vi "MultiAxisControl.vi"() -> ()   [LabVIEW 2018, in "Aerotech.lvlib"]
uses:
  Aerotech.lvlib
  Parameters/GetAxisParameterDouble.vi
  Motion/AbortSingle.vi
  Parameters/GetAxisParameterString.vi
  Motion/MoveIncSingle.vi
  Motion/FreerunSingle.vi
  Motion/FaultAckSingle.vi
  Motion/HomeSingle.vi
  Motion/DisableSingle.vi
  Motion/EnableSingle.vi
  Utility/AxisControl.ctl
panel:
  in  "Disconnect?":bool
  in  "Show First":i32=2 caption="Axes" min=0 max=32
  out "Status":string
  in  "StopProgram":bool caption="Stop"
  out "do stop":bool
  in  "stop":bool
  out "Error":string
  in  "Init":bool=TRUE
  in  "Abort Motion":bool
  in  "Reset Controller":bool
  in  "In Task:":i32(ring)=1 items=["TLibrary", "T01", "T02", "T03", "T04", "T05", "T06", "T07", "T08", "T09", "T10", "T11", "T12", "T13", "T14", "T15", "T16", "T17", "T18", "T19", "T20", "T21", "T22", "T23", "T24", "T25", "T26", "T27", "T28", "T29", "T30", "T31"]
  in  "ExecuteProgram":bool caption="Execute"
  in  "Program:":path
  in  "Axes":T1[](array[typedef])
  in  "Status":string
  in  "Execute":bool
  in  "Command:":string
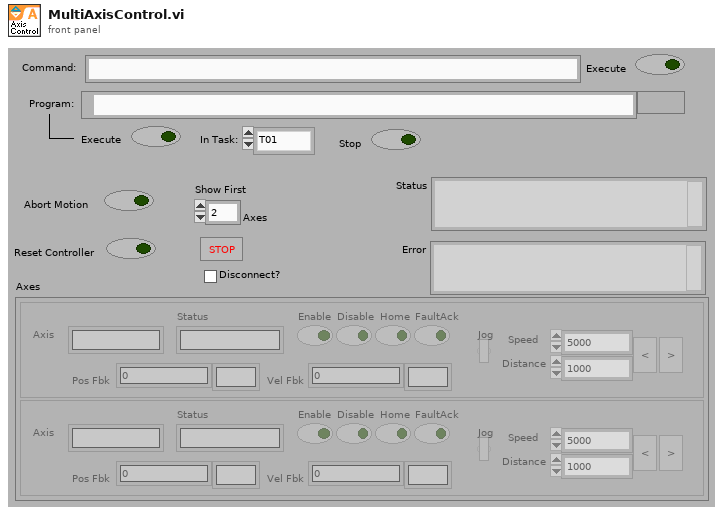
[diagram p1: front panel]
types:
  T1 = typedef "Aerotech.lvlib/AxisControl.ctl" = cluster{"Axis":string, "Enable":bool, "Disable":bool, "Home":bool, "FaultAck":bool, "Jog":bool, "Speed":dbl, "Distance":dbl, "Jog Left":bool, "Jog Right":bool, "Status":string, "Pos Fbk":dbl, "Vel Fbk":dbl, "Pos Units":string, "Vel Units":string}
  T2 = cluster{"new reference":refnum<k24>, "Event Callback":refnum<k27>, "ControllerDiagPacket":refnum<user-event>, "Event Registration Refnum":refnum<event-registration>}
  T3 = enum32{"invalid app kind", "Development System", "Run Time System", "Student Edition", "Embedded LabVIEW", "Evaluation", "Custom"}
  T4 = cluster{"Axis":string, "Enable":bool, "Disable":bool, "Home":bool, "FaultAck":bool, "Jog":bool, "Speed":dbl, "Distance":dbl, "Jog Left":bool, "Jog Right":bool, "Status":string, "Pos Fbk":dbl, "Vel Fbk":dbl, "Pos Units":string, "Vel Units":string}
  T5 = typedef "AxisDiagPacket.ctl" = cluster{"Axis Name":string, "Analog Input 0":dbl, "Analog Input 1":dbl, "Axis Fault (num)":i32, "Axis Fault (str)":string, "Axis Fault (bits)":cluster{"AmplifierFault":bool, "AmplifierTemperatureFault":bool, "CcwEndOfTravelLimitFault":bool, "CcwSoftwareLimitFault":bool, "CommunicationLostFault":bool, "CwEndOfTravelLimitFault":bool, "CwSoftwareLimitFault":bool, "EmergencyStopFault":bool, "EncoderFault":bool, "ExternalFault":bool, "FeedbackScalingFault":bool, "GantryMisalignFault ":bool, "HallSensorFault":bool, "InPositionTimeoutFault":bool, "MarkerSearchFault":bool, "MaxVelocityCommandFault":bool, "MissedInterruptFault":bool, "MotorTemperatureFault":bool, "None":bool, "OverCurrentFault":bool, "PositionErrorFault":bool, "PositionFeedbackFault":bool, "PowerSupplyFault":bool, "ProbeInputFault":bool, "SafeZoneFault":bool, "VelocityErrorFault":bool, "VelocityFeedbackFault":bool, "VoltageClampFault":bool, "InternalFault":bool}, "Axis Status (num)":i32, "Axis Status (str)":string, "Axis Status (bits)":cluster{"BacklashActive":bool, "CalibrationEnabled1D":bool, "CalibrationEnabled2D":bool, "CommandValid":bool, "DriveAbortPending":bool, "DrivePending":bool, "Enabling":bool, "GainMappingEnabled":bool, "GantryAligned":bool, "GantryRealigning":bool, "Homed":bool, "Homing":bool, "IFOVEnabled":bool, "JogGenerating":bool, "Jogging":bool, "JoystickControl":bool, "MasterSlaveControl":bool, "MotionBlocked":bool, "MotionClamped":bool, "MoveDone":bool, "None":bool, "NotVirtual":bool, "Profiling":bool, "Stability0":bool, "Stability1":bool, "TrajectoryFiltering":bool, "WaitDone":bool}, "Current Command":sgl, "Current Error":sgl, "Current Feedback":sgl, "Digital Inputs":i32, "Digital Outputs":i32, "Drive Status":i32, "Drive Status (str)":string, "Drive Status (bits)":cluster{"AccelerationPhase":bool, "AutofocusActive":bool, "BrakeOutput":bool, "CcwEndOfTravelLimitInput":bool, "CosineEncoderError":bool, "CurrentClamp":bool, "CwEndOfTravelLimitInput":bool, "DecelerationPhase":bool, "DualLoopActive":bool, "EmergencyStopInput":bool, "Enabled":bool, "EncoderClipping":bool, "GalvoCalibrationEnabled":bool, "GalvoPowerCorrection":bool, "HallAInput":bool, "HallBInput":bool, "HallCInput":bool, "HighResolutionMode":bool, "HomeLimitInput":bool, "InPosition":bool, "InPosition2":bool, "MarkerInput":bool, "MarkerLatch":bool, "MoveActive":bool, "NoMotorSupply":bool, "None":bool, "PowerLimiting":bool, "ProgrammingFlash":bool, "ProgrammingMXH":bool, "PSOHaltLatch":bool, "ServoControl":bool, "SineEncoderError":bool}, "Position Feedback Auxiliary":dbl, "Position Command":dbl, "Position Error":dbl, "Position Feedback":dbl, "Program Position Command":dbl, "Program Position Error":dbl, "Program Position Feedback":dbl, "Velocity Command":dbl, "Velocity Error":dbl, "Velocity Feedback":dbl}
  T6 = cluster{"Axis":string, "Enable":bool, "Disable":bool, "Home":bool, "FaultAck":bool, "Jog":bool, "Speed":dbl, "Distance":dbl, "Jog Left":bool, "Jog Right":bool, "Status":string, "Pos Fbk":dbl, "Vel Fbk":dbl, "Pos Units":string, "Vel Units":string}[]
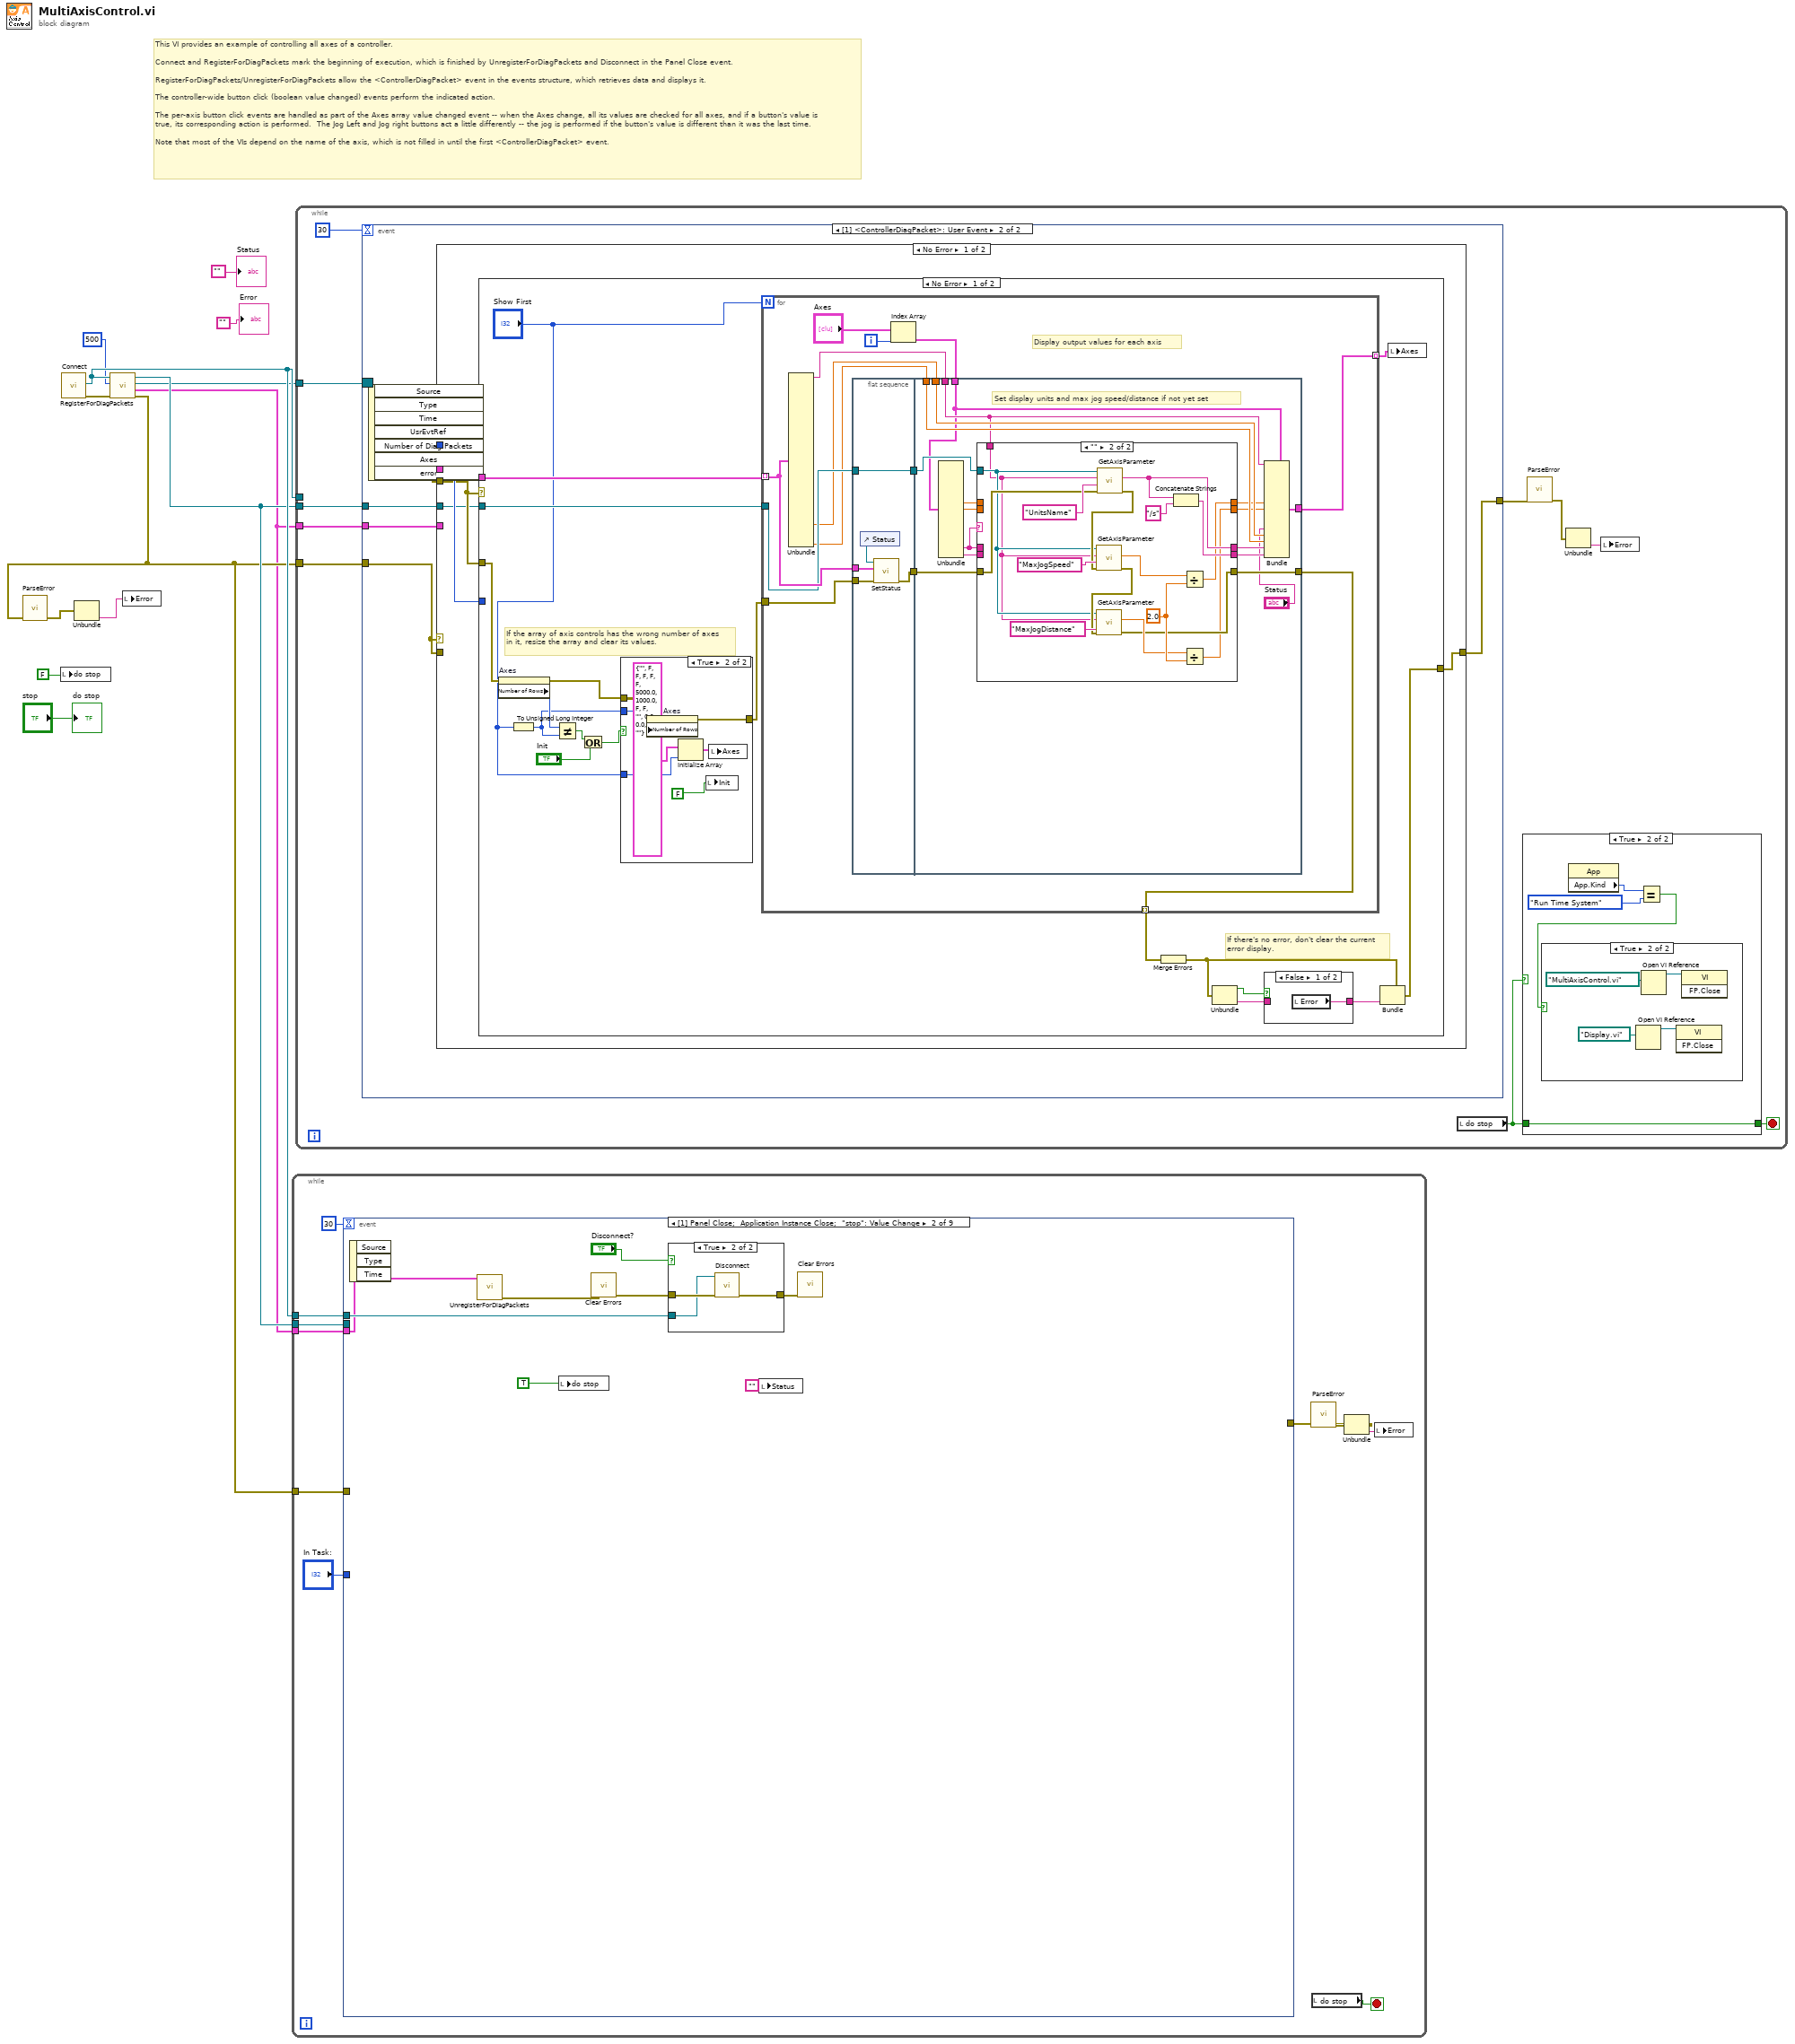
[diagram p0: block diagram]
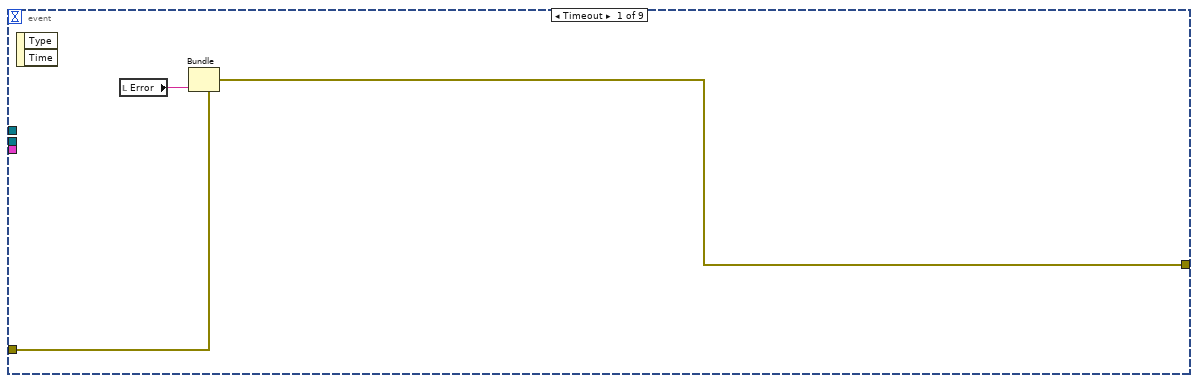
[diagram p2: hidden frame]
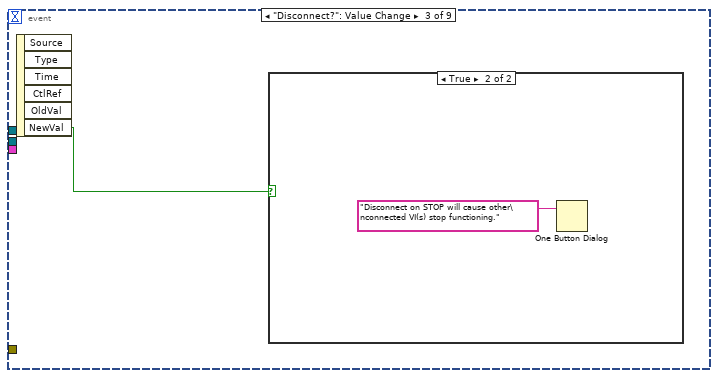
[diagram p4: hidden frame]
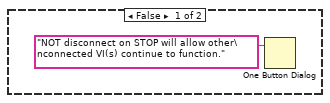
[diagram p5: hidden frame]
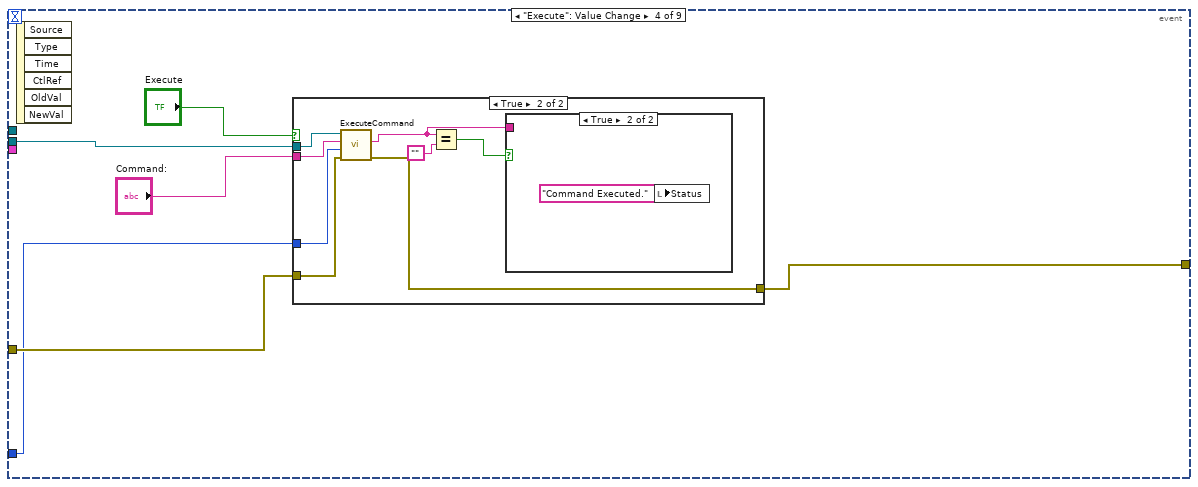
[diagram p6: hidden frame]
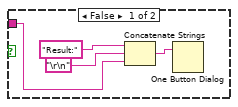
[diagram p8: hidden frame]
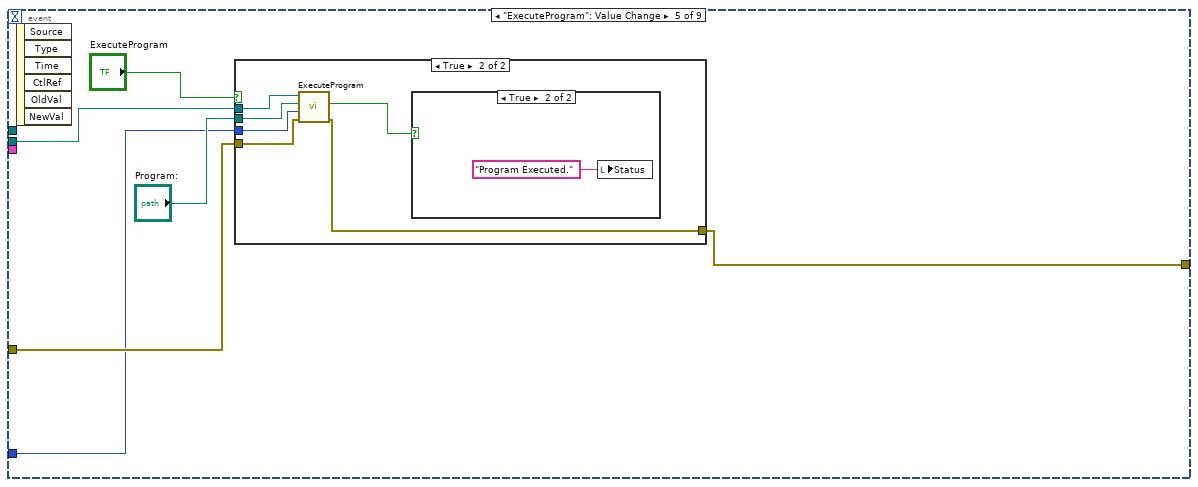
[diagram p9: hidden frame]
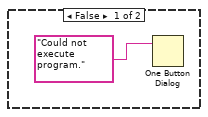
[diagram p11: hidden frame]
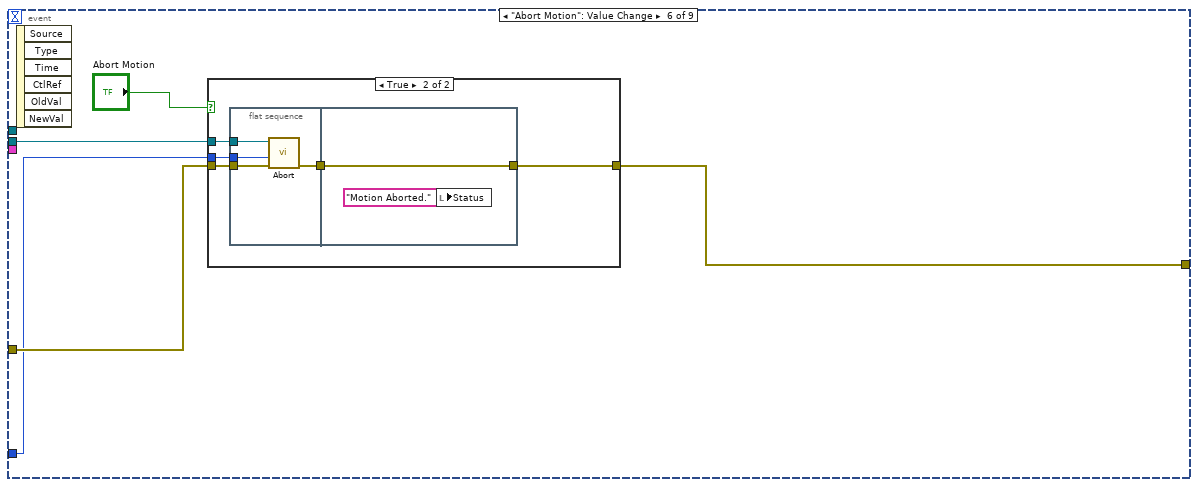
[diagram p12: hidden frame]
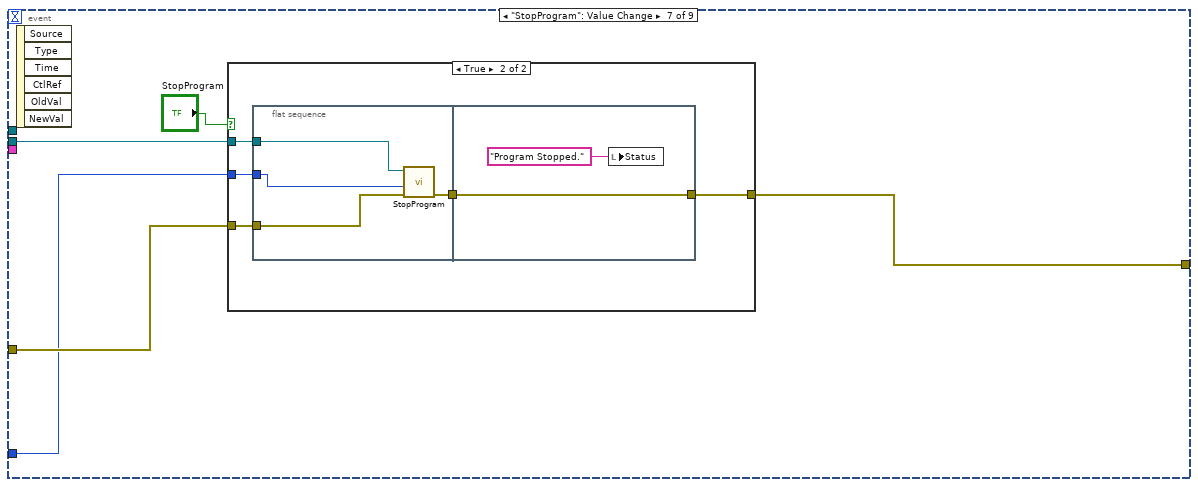
[diagram p14: hidden frame]
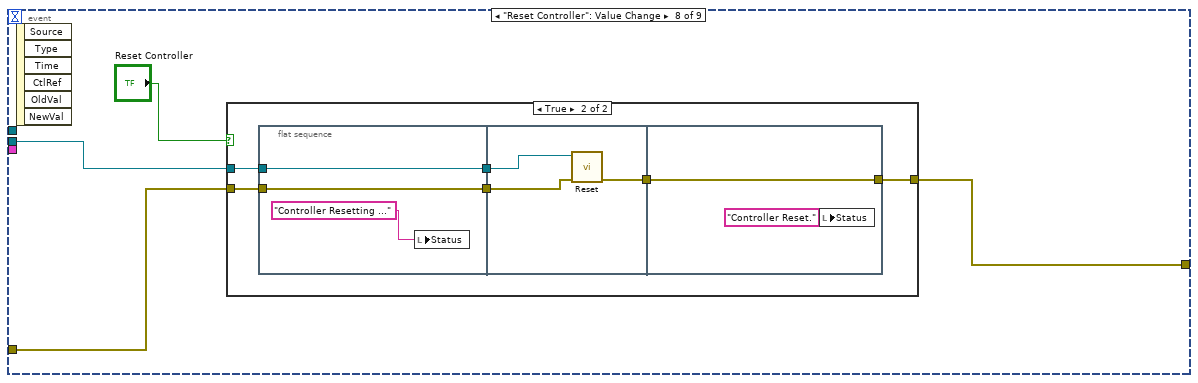
[diagram p16: hidden frame]
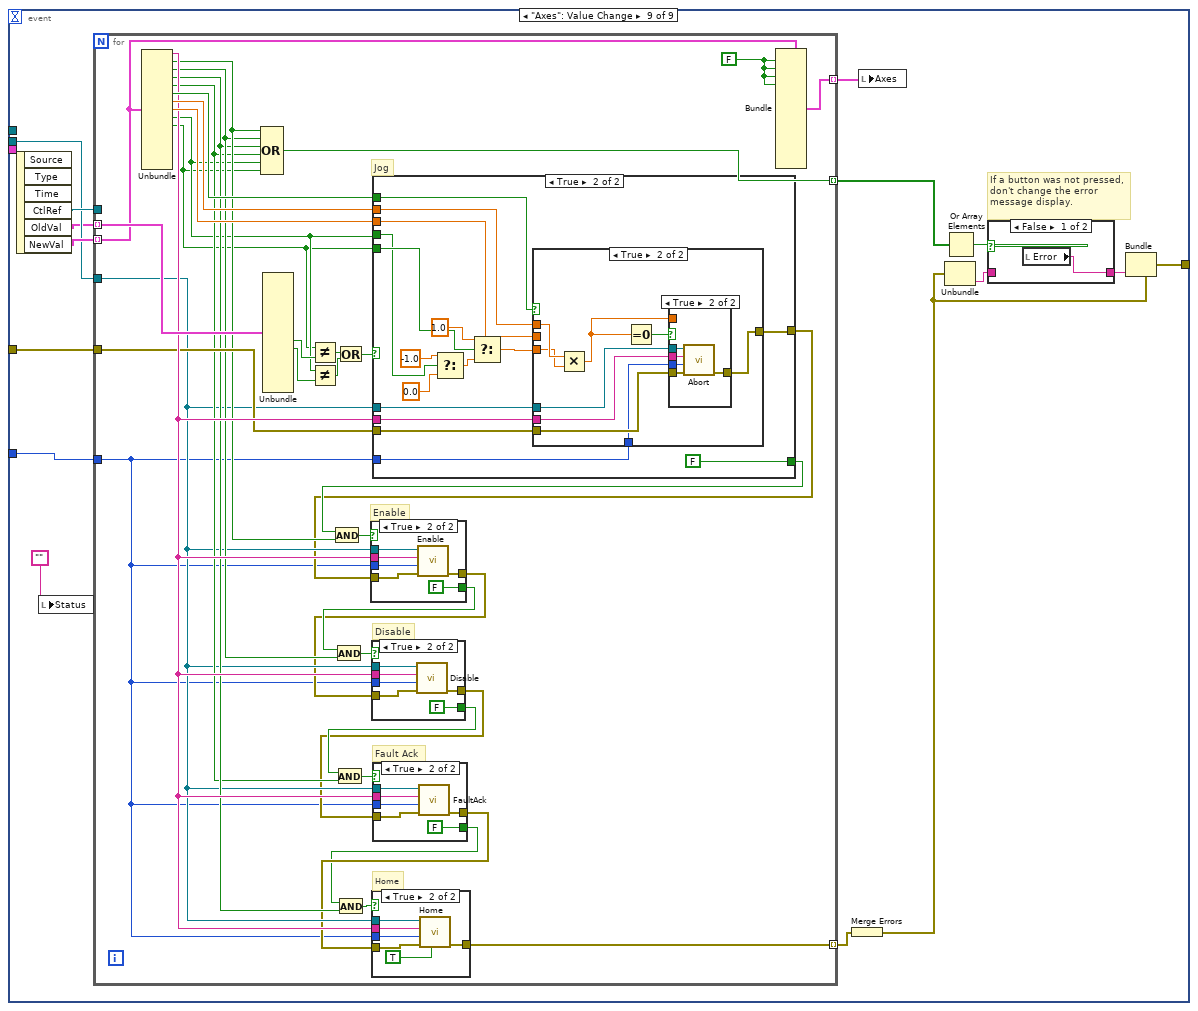
[diagram p18: hidden frame]
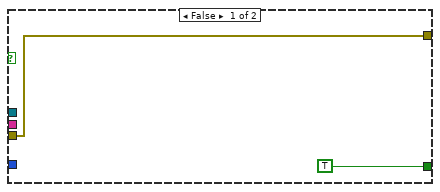
[diagram p20: hidden frame]
diagram:
  # "This VI provides an example of controlling all axes of a controller. \n\nConnect and RegisterForDiagPackets mark the beginning of execution, which is finished by UnregisterForDiagPackets and Disconnect in the Panel Close event.\n\nRegisterForDiagPackets/UnregisterForDiagPackets allow the <ControllerDiagPacket> event in the events structure, which retrieves data and displays it.\n\nThe controller-wide button click (boolean value changed) events perform the indicated action.\n\nThe per-axis button click events are handled as part of the Axes array value changed event -- when the Axes change, all its values are checked for all axes, and if a button's value is true, its corresponding action is performed.  The Jog Left and Jog right buttons act a little differently -- the jog is performed if the button's value is different than it was the last time.\n\nNote that most of the VIs depend on the name of the axis, which is not filled in until the first <ControllerDiagPacket> event."
  n1 = local write "do stop"(FALSE ("do stop")) -> ()
  n2 = call "Connect.vi"() -> ("error out"=w7:errorcluster, "controller"=w6:refnum<k24>)  [unwired: 10 in]
  n3 = call "RegisterForDiagPackets.vi"("error in (no error)"=w7, "refresh interval (default)"=500, "Controller in"=w6) -> ("error out"=w3:errorcluster, "Event Metadata"=w2:T2, "Event Registration Refnum"=w4:refnum<event-registration>, "Controller out"=w5:refnum<k24>)  [unwired: 4 in]
  n4 = call "ParseError.vi"("error in (no error)"=w3) -> ("error out"=w11:errorcluster)  [unwired: 10 in]
  n5 = Unbundle(w11) -> ("source"=w12:string)  [unwired: 2 out]
  n6 = local write "Error"(w12) -> ()
  n7 = while {
    tunnel: w6 -> [w19]
    tunnel: w5 -> [w18]
    tunnel: w3 -> [w17]
    tunnel: w2 -> [w14]
    stop <- w16 stop-if-true
    n8 = event shown="[1] Panel Close;  Application Instance Close;  \"stop\": Value Change" {
      selector: _ -> [_ _ _ _ _ _ _ _ _]
      dyn-events: _ -> [_ _ _ _ _ _ _ _ _]
      timeout: 30 -> [_ _ _ _ _ _ _ _ _]
      tunnel: w18 -> [_ _ _ w46 w66 w80 w95 w113 w142]
      tunnel: w17 -> [w26 _ _ w45 w64 w81 w97 w112 w141]
      tunnel: [w25 _ _ w43 w63 w78 w96 w111 w136] -> w21
      tunnel: w19 -> [_ w33 _ _ _ _ _ _ _]
      tunnel: "In Task:" -> [_ _ _ w42 w62 w77 w94 _ w130]
      tunnel: w14 -> [_ w27 _ _ _ _ _ _ _]
      event Timeout {
        n9 = event-data() -> ()  [unwired: 1 in, 2 out]
        n10 = local read "Error"() -> (w24:string)
        n11 = Bundle(cluster=w26, "source"=w24) -> (w25:errorcluster)  [unwired: 2 in]
      }
      event Panel Close; Application Instance Close; "stop": Value Change {
        n12 = event-data() -> ()  [unwired: 1 in, 3 out]
        n13 = call "UnregisterForDiagPackets.vi"("Event Metadata"=w27) -> ("error out"=w28:errorcluster)  [unwired: 9 in]
        n14 = local write "do stop"(TRUE) -> ()
        n15 = call <vilib>:"Clear Errors.vi"("error in (no error)"=w28) -> ("error out"=w34:errorcluster)  [unwired: 5 in, 1 out]
        n16 = case shown="True" "Disconnect?" {
          tunnel: w34 -> [w35 w38]
          tunnel: w33 -> [_ w37]
          tunnel: [w35 w36] -> w32
          frame False {
          }
          frame True {
            n17 = call "Disconnect.vi"("error in (no error)"=w38, "controller"=w37) -> ("error out"=w36:errorcluster)  [unwired: 9 in]
          }
        }
        n18 = local write "Status"("") -> ()
        n19 = call <vilib>:"Clear Errors.vi"("error in (no error)"=w32) -> ()  [unwired: 5 in, 2 out]
      }
      event "Disconnect?": Value Change {
        n20 = event-data() -> ("NewVal"=w39:bool)  [unwired: 1 in, 5 out]
        n21 = case shown="True" w39 {
          frame False {
            n22 = One Button Dialog(message="NOT disconnect on STOP will allow other\nconnected VI(s) continue to function.") -> ()  [unwired: 1 in, 1 out]
          }
          frame True {
            n23 = One Button Dialog(message="Disconnect on STOP will cause other\nconnected VI(s) stop functioning.") -> ()  [unwired: 1 in, 1 out]
          }
        }
      }
      event "Execute": Value Change {
        n24 = event-data() -> ()  [unwired: 1 in, 6 out]
        n25 = case shown="True" "Execute" {
          tunnel: w46 -> [_ w56]
          tunnel: w45 -> [w48 w54]
          tunnel: "Command:" -> [_ w55]
          tunnel: [w48 w50] -> w43
          tunnel: w42 -> [_ w49]
          frame False {
          }
          frame True {
            n26 = call "ExecuteCommand.vi"("error in (no error)"=w54, "taskId"=w49, "Command Code"=w55, "controller in"=w56) -> ("error out"=w50:errorcluster, "return value"=w51:string)  [unwired: 5 in, 1 out]
            n27 = Equal?(x=w51, y="") -> (x = y?=w52:bool)
            n28 = case shown="True" w52 {
              tunnel: w51 -> [w57 _]
              frame False {
                n29 = Concatenate Strings("Result:", "\r\n", w57) -> (w60:string)
                n30 = One Button Dialog(message=w60) -> ()  [unwired: 1 in, 1 out]
              }
              frame True {
                n31 = local write "Status"("Command Executed." ("Status")) -> ()
              }
            }
          }
        }
      }
      event "ExecuteProgram": Value Change {
        n32 = event-data() -> ()  [unwired: 1 in, 6 out]
        n33 = case shown="True" "ExecuteProgram" {
          tunnel: w66 -> [_ w74]
          tunnel: w64 -> [w68 w72]
          tunnel: "Program:" -> [_ w73]
          tunnel: w62 -> [_ w70]
          tunnel: [w68 w69] -> w63
          frame False {
          }
          frame True {
            n34 = call "ExecuteProgram.vi"("error in (no error)"=w72, "taskId"=w70, "program name and path"=w73, "controller in"=w74) -> ("error out"=w69:errorcluster, "success"=w71:bool)  [unwired: 5 in, 1 out]
            n35 = case shown="True" w71 {
              frame False {
                n36 = One Button Dialog(message="Could not execute program.") -> ()  [unwired: 1 in, 1 out]
              }
              frame True {
                n37 = local write "Status"("Program Executed." ("Status")) -> ()
              }
            }
          }
        }
      }
      event "Abort Motion": Value Change {
        n38 = event-data() -> ()  [unwired: 1 in, 6 out]
        n39 = case shown="True" "Abort Motion" {
          tunnel: w80 -> [_ w87]
          tunnel: w81 -> [w82 w86]
          tunnel: [w82 w85] -> w78
          tunnel: w77 -> [_ w83]
          frame False {
          }
          frame True {
            n40 = flat-sequence {
              tunnel: w87 -> [w91]
              tunnel: w86 -> [w90]
              tunnel: [w89] -> w84
              tunnel: w83 -> [w88]
              tunnel: [w93] -> w85
              tunnel: w84 -> [w93]
              frame #0 {
                n41 = call-poly "Abort.vi"("error in (no error)"=w90, "taskId"=w88, "controller in"=w91) -> ("error out"=w89:errorcluster)  [unwired: 7 in, 1 out]
              }
              frame #1 {
                n42 = local write "Status"("Motion Aborted." ("Status")) -> ()
              }
            }
          }
        }
      }
      event "StopProgram": Value Change {
        n43 = event-data() -> ()  [unwired: 1 in, 6 out]
        n44 = case shown="True" "StopProgram" {
          tunnel: w97 -> [w99 w104]
          tunnel: [w99 w103] -> w96
          tunnel: w95 -> [_ w102]
          tunnel: w94 -> [_ w100]
          frame False {
          }
          frame True {
            n45 = flat-sequence {
              tunnel: w104 -> [w108]
              tunnel: w102 -> [w106]
              tunnel: [w107] -> w101
              tunnel: w100 -> [w105]
              tunnel: [w110] -> w103
              tunnel: w101 -> [w110]
              frame #0 {
                n46 = call "StopProgram.vi"("error in (no error)"=w108, "taskId"=w105, "controller in"=w106) -> ("error out"=w107:errorcluster)  [unwired: 7 in, 1 out]
              }
              frame #1 {
                n47 = local write "Status"("Program Stopped." ("Status")) -> ()
              }
            }
          }
        }
      }
      event "Reset Controller": Value Change {
        n48 = event-data() -> ()  [unwired: 1 in, 6 out]
        n49 = case shown="True" "Reset Controller" {
          tunnel: w113 -> [_ w121]
          tunnel: w112 -> [w115 w120]
          tunnel: [w115 w119] -> w111
          frame False {
          }
          frame True {
            n50 = flat-sequence {
              tunnel: w120 -> [w123]
              tunnel: w121 -> [w124]
              tunnel: [w124] -> w118
              tunnel: [w123] -> w117
              tunnel: w118 -> [w127]
              tunnel: w117 -> [w126]
              tunnel: [w125] -> w116
              tunnel: [w129] -> w119
              tunnel: w116 -> [w129]
              frame #0 {
                n51 = local write "Status"("Controller Resetting ..." ("Errors")) -> ()
              }
              frame #1 {
                n52 = call "Reset.vi"("error in (no error)"=w126, "controller in"=w127) -> ("error out"=w125:errorcluster)  [unwired: 8 in, 1 out]
              }
              frame #2 {
                n53 = local write "Status"("Controller Reset." ("Status")) -> ()
              }
            }
          }
        }
      }
      event "Axes": Value Change {
        # "If a button was not pressed, don't change the error message display."
        n54 = event-data() -> ("CtlRef"=w143:refnum<vi>, "OldVal"=w140:T1[], "NewVal"=w144:T1[])  [unwired: 1 in, 3 out]
        n55 = local write "Status"("") -> ()
        n56 = for {
          tunnel: w144 -> [w166] mode=indexing
          tunnel: w143 -> [_]
          tunnel: w142 -> [w164]
          tunnel: w141 -> [w172]
          tunnel: w140 -> [w179] mode=indexing
          tunnel: [w153] -> w139 mode=indexing
          tunnel: [w149] -> w138 mode=indexing
          tunnel: [w167] -> w133 mode=indexing
          tunnel: w130 -> [w147]
          w148 = FALSE
          # "Jog"
          # "Fault Ack"
          # "Home"
          # "Disable"
          # "Enable"
          n57 = Unbundle(w166) -> ("Axis"=w173:string, "Enable"=w171:bool, "Disable"=w170:bool, "Home"=w169:bool, "FaultAck"=w168:bool, "Jog"=w180:bool, "Speed"=w182:dbl, "Distance"=w181:dbl, "Jog Left"=w165:bool, "Jog Right"=w154:bool)  [unwired: 5 out]
          n58 = Compound Arithmetic op=OR(w171, w170, w169, w168, w165, w154) -> (w149:bool)
          n59 = Unbundle(w179) -> ("Jog Left"=w175:bool, "Jog Right"=w174:bool)  [unwired: 13 out]
          n60 = Not Equal?(x=w154, y=w175) -> (x != y?=w177:bool)
          n61 = Not Equal?(x=w165, y=w174) -> (x != y?=w176:bool)
          n62 = Or(x=w177, y=w176) -> (x .or. y?=w178:bool)
          n63 = case shown="True" w178 {
            tunnel: w180 -> [_ w195]
            tunnel: w182 -> [_ w193]
            tunnel: w181 -> [_ w194]
            tunnel: w154 -> [_ w189]
            tunnel: w165 -> [_ w188]
            tunnel: w164 -> [_ w192]
            tunnel: w173 -> [_ w191]
            tunnel: w172 -> [w184 w190]
            tunnel: [w184 w187] -> w157
            tunnel: [TRUE FALSE] -> w162
            tunnel: w147 -> [_ w185]
            frame False {
            }
            frame True {
              n64 = Select(t=-1.0, s=w188, f=0.0) -> (s? t:f=w200:dbl)
              n65 = Select(t=1.0, s=w189, f=w200) -> (s? t:f=w196:dbl)
              n66 = case shown="True" w195 {
                tunnel: w193 -> [w204 w218]
                tunnel: w194 -> [w209 _]
                tunnel: w196 -> [w208 w217]
                tunnel: w190 -> [w207 w216]
                tunnel: w191 -> [w203 w215]
                tunnel: w192 -> [w202 w214]
                tunnel: [w206 w213] -> w187
                tunnel: w185 -> [w201 w212]
                frame False {
                  n67 = Multiply(x=w209, y=w208) -> (x*y=w205:dbl)
                  n68 = call-poly "MoveInc.vi"("distance"=w205, "speed"=w204, "error in (no error)"=w207, "taskId"=w201, "axis name"=w203, "controller in"=w202) -> ("error out"=w206:errorcluster)  [unwired: 4 in, 1 out]
                }
                frame True {
                  n69 = Multiply(x=w218, y=w217) -> (x*y=w210:dbl)
                  n70 = Equal To 0?(x=w210) -> (x = 0?=w211:bool)
                  n71 = case shown="True" w211 {
                    tunnel: w216 -> [w224 w229]
                    tunnel: w215 -> [w223 w226]
                    tunnel: w214 -> [w222 w227]
                    tunnel: [w221 w228] -> w213
                    tunnel: w210 -> [w220 _]
                    tunnel: w212 -> [w219 w225]
                    frame False {
                      n72 = call-poly "Freerun.vi"("speed"=w220, "error in (no error)"=w224, "taskId"=w219, "axis name"=w223, "controller in"=w222) -> ("error out"=w221:errorcluster)  [unwired: 5 in, 1 out]
                    }
                    frame True {
                      n73 = call-poly "Abort.vi"("error in (no error)"=w229, "taskId"=w225, "axis name? (all)"=w226, "controller in"=w227) -> ("error out"=w228:errorcluster)  [unwired: 6 in, 1 out]
                    }
                  }
                }
              }
            }
          }
          n74 = And(x=w162, y=w171) -> (x .and. y?=w163:bool)
          n75 = case shown="True" w163 {
            tunnel: w164 -> [_ w260]
            tunnel: w157 -> [w254 w259]
            tunnel: w173 -> [_ w257]
            tunnel: [w254 w258] -> w156
            tunnel: [TRUE FALSE] -> w160
            tunnel: w147 -> [_ w255]
            frame False {
            }
            frame True {
              n76 = call-poly "Enable.vi"("error in (no error)"=w259, "taskId"=w255, "axis name"=w257, "controller in"=w260) -> ("error out"=w258:errorcluster)  [unwired: 6 in, 1 out]
            }
          }
          n77 = And(x=w160, y=w170) -> (x .and. y?=w161:bool)
          n78 = case shown="True" w161 {
            tunnel: w164 -> [_ w252]
            tunnel: w156 -> [w246 w250]
            tunnel: w173 -> [_ w251]
            tunnel: [w246 w249] -> w155
            tunnel: [TRUE FALSE] -> w158
            tunnel: w147 -> [_ w247]
            frame False {
            }
            frame True {
              n79 = call-poly "Disable.vi"("error in (no error)"=w250, "taskId"=w247, "axis name"=w251, "controller in"=w252) -> ("error out"=w249:errorcluster)  [unwired: 6 in, 1 out]
            }
          }
          n80 = And(x=w158, y=w168) -> (x .and. y?=w159:bool)
          n81 = case shown="True" w159 {
            tunnel: w164 -> [_ w237]
            tunnel: w155 -> [w231 w235]
            tunnel: w173 -> [_ w236]
            tunnel: [w231 w234] -> w152
            tunnel: [TRUE FALSE] -> w150
            tunnel: w147 -> [_ w232]
            frame False {
            }
            frame True {
              n82 = call-poly "FaultAck.vi"("error in (no error)"=w235, "taskId"=w232, "axis name"=w236, "controller in"=w237) -> ("error out"=w234:errorcluster)  [unwired: 6 in, 1 out]
            }
          }
          n83 = And(x=w150, y=w169) -> (x .and. y?=w151:bool)
          n84 = case shown="True" w151 {
            tunnel: w164 -> [_ w244]
            tunnel: w173 -> [_ w243]
            tunnel: w152 -> [w238 w242]
            tunnel: [w238 w241] -> w153
            tunnel: w147 -> [_ w239]
            frame False {
            }
            frame True {
              n85 = call-poly "Home.vi"("return immediately"=TRUE ("Return Immediately ?"), "error in (no error)"=w242, "taskId"=w239, "axis name"=w243, "controller in"=w244) -> ("error out"=w241:errorcluster)  [unwired: 5 in, 1 out]
            }
          }
          n86 = Bundle(cluster=w166, "Enable"=w148, "Disable"=w148, "Home"=w148, "FaultAck"=w148) -> (w167:T1)  [unwired: 11 in]
        }
        n87 = Merge Errors(w139) -> (w132:errorcluster)
        n88 = local write "Axes"(w133) -> ()
        n89 = Unbundle(w132) -> ("source"=w135:string)  [unwired: 2 out]
        n90 = Or Array Elements(Boolean array=w138) -> (logical OR=w137:bool)
        n91 = case shown="False" w137 {
          tunnel: w135 -> [_ w146]
          tunnel: [w145 w146] -> w134
          frame False {
            n92 = local read "Error"() -> (w145:string)
          }
          frame True {
          }
        }
        n93 = Bundle(cluster=w132, "source"=w134) -> (w136:errorcluster)  [unwired: 2 in]
      }
    }
    n94 = call "ParseError.vi"("error in (no error)"=w21) -> ("error out"=w23:errorcluster)  [unwired: 10 in]
    n95 = local read "do stop"() -> (w16:bool)
    n96 = Unbundle(w23) -> ("source"=w22:string)  [unwired: 2 out]
    n97 = local write "Error"(w22) -> ()
  }
  n98 = while {
    tunnel: w4 -> [w267]
    tunnel: w5 -> [w265]
    tunnel: w6 -> [_]
    tunnel: w3 -> [w264]
    tunnel: w2 -> [w263]
    stop <- w262 stop-if-true
    n99 = event shown="[1] <ControllerDiagPacket>: User Event" {
      selector: w267 -> [_ _]
      dyn-events: _ -> [_ _]
      timeout: 30 -> [_ _]
      tunnel: [w280 w289] -> w266
      tunnel: w265 -> [_ w288]
      tunnel: w264 -> [w282 w287]
      tunnel: w263 -> [_ w283]
      event Timeout {
        n100 = event-data() -> ()  [unwired: 1 in, 2 out]
        n101 = local read "Error"() -> (w281:string)
        n102 = Bundle(cluster=w282, "source"=w281) -> (w280:errorcluster)  [unwired: 2 in]
      }
      event User Event {
        n103 = event-data() -> ("Number of Diag Packets"=w286:i32, "Axes"=w285:T5[], "error"=w284:errorcluster)  [unwired: 1 in, 4 out]
        n104 = case shown="No Error" w287 {
          tunnel: w285 -> [w294 _]
          tunnel: [w293 w381] -> w289
          tunnel: w286 -> [w292 _]
          tunnel: w284 -> [w291 _]
          tunnel: w287 -> [_ w381]
          tunnel: w288 -> [w290 _]
          tunnel: w283 -> [_ _]
          frame No Error {
            n105 = case shown="No Error" w291 {
              tunnel: w294 -> [w312 _]
              tunnel: [w302 w380] -> w293
              tunnel: w291 -> [w298 w380]
              tunnel: w292 -> [_ _]
              tunnel: w290 -> [w296 _]
              frame No Error {
                # "If there's no error, don't clear the current error display."
                # "If the array of axis controls has the wrong number of axes in it, resize the array and clear its values."
                n106 = property on="Axes" class="Arr (strict)"(error in=w298) -> (error out=w297:errorcluster, "Number of Rows"=w308:u32)  [unwired: 1 in, 1 out]
                n107 = To Unsigned Long Integer(number="Show First") -> (unsigned 32bit integer=w307:u32)
                n108 = Not Equal?(x=w308, y=w307) -> (x != y?=w306:bool)
                n109 = Or(x=w306, y="Init") -> (x .or. y?=w305:bool)
                n110 = case shown="True" w305 {
                  tunnel: w297 -> [w372 w379]
                  tunnel: [w372 w378] -> w311
                  tunnel: w307 -> [_ w374]
                  tunnel: "Show First" -> [_ w375]
                  frame False {
                  }
                  frame True {
                    n111 = property on="Axes" class="Arr (strict)"(error in=w379, "Number of Rows"=w374) -> (error out=w378:errorcluster)  [unwired: 1 in, 1 out]
                    n112 = Initialize Array(T4 {"Axis"="", "Enable"=FALSE, "Disable"=FALSE, "Home"=FALSE, "FaultAck"=FALSE, "Jog"=FALSE, "Speed"=5000.0, "Distance"=1000.0, "Jog Left"=FALSE, "Jog Right"=FALSE, "Status"="", "Pos Fbk"=0.0, "Vel Fbk"=0.0, "Pos Units"="", "Vel Units"=""} ("Axis"), w375) -> (w377:T6)
                    n113 = local write "Init"(FALSE ("Init")) -> ()
                    n114 = local write "Axes"(w377) -> ()
                  }
                }
                n115 = for {
                  N: "Show First" -> [_]
                  tunnel: w311 -> [w326]
                  tunnel: w312 -> [w327] mode=indexing
                  tunnel: [w325] -> w310 mode=indexing
                  tunnel: [w320] -> w309 mode=indexing
                  tunnel: w296 -> [w318]
                  i -> [w321]
                  # "Display output values for each axis"
                  n116 = Unbundle(w327) -> ("Axis Name"=w324:string, "Program Position Feedback"=w316:dbl, "Velocity Feedback"=w315:dbl)  [unwired: 24 out]
                  n117 = flat-sequence {
                    tunnel: w327 -> [w331]
                    tunnel: w326 -> [w330]
                    tunnel: [w329] -> w319
                    tunnel: w318 -> [w328]
                    tunnel: [w328] -> w317
                    tunnel: w322 -> [w342]
                    tunnel: w324 -> [w344]
                    tunnel: w316 -> [w348]
                    tunnel: w315 -> [w347]
                    tunnel: w319 -> [w345]
                    tunnel: w317 -> [w343]
                    tunnel: [w349] -> w325
                    tunnel: [w346] -> w320
                    frame #0 {
                      n118 = control-ref of="Status"() -> (w332:refnum<vi>)
                      n119 = call "SetStatus.vi"("error in (no error)"=w330, "AxisDiagPacket"=w331, "Status string"=w332) -> ("error out"=w329:errorcluster)  [unwired: 8 in]
                    }
                    frame #1 {
                      # "Set display units and max jog speed/distance if not yet set"
                      n120 = Unbundle(w342) -> ("Speed"=w337:dbl, "Distance"=w336:dbl, "Pos Units"=w341:string, "Vel Units"=w340:string)  [unwired: 11 out]
                      n121 = case shown="\"\"" w341 {
                        tunnel: w343 -> [_ w356]
                        tunnel: [w354 w359] -> w346
                        tunnel: w345 -> [w354 w369]
                        tunnel: w344 -> [_ w355]
                        tunnel: w341 -> [w352 _]
                        tunnel: w340 -> [w353 _]
                        tunnel: [w353 w368] -> w339
                        tunnel: [w352 w367] -> w338
                        tunnel: w337 -> [w351 _]
                        tunnel: w336 -> [w350 _]
                        tunnel: [w351 w358] -> w335
                        tunnel: [w350 w357] -> w334
                        frame Default {
                        }
                        frame "" {
                          w366 = 2.0 ("y")
                          n122 = call-poly "GetAxisParameter.vi"("error in (no error)"=w369, "Parameter Name"="UnitsName" ("parameter name"), "axis name"=w355, "controller in"=w356) -> ("error out"=w360:errorcluster, "value"=w367:string)  [unwired: 5 in, 1 out]
                          n123 = call-poly "GetAxisParameter.vi"("error in (no error)"=w360, "Parameter Name"="MaxJogSpeed" ("parameter name"), "axis name"=w355, "controller in"=w356) -> ("error out"=w361:errorcluster, "value"=w364:dbl)  [unwired: 5 in, 1 out]
                          n124 = call-poly "GetAxisParameter.vi"("error in (no error)"=w361, "Parameter Name"="MaxJogDistance" ("parameter name"), "axis name"=w355, "controller in"=w356) -> ("error out"=w359:errorcluster, "value"=w365:dbl)  [unwired: 5 in, 1 out]
                          n125 = Concatenate Strings(w367, "/s" ("string")) -> (w368:string)
                          n126 = Divide(x=w364, y=w366) -> (x/y=w358:dbl)
                          n127 = Divide(x=w365, y=w366) -> (x/y=w357:dbl)
                        }
                      }
                      n128 = Bundle(cluster=w342, "Axis"=w344, "Speed"=w335, "Distance"=w334, "Status"="Status", "Pos Fbk"=w348, "Vel Fbk"=w347, "Pos Units"=w338, "Vel Units"=w339) -> (w349:T1)  [unwired: 7 in]
                    }
                  }
                  n129 = Index Array(array="Axes", index=w321) -> (element=w322:T1)
                }
                n130 = Merge Errors(w309) -> (w303:errorcluster)
                n131 = Unbundle(w303) -> ("status"=w301:bool, "source"=w300:string)  [unwired: 1 out]
                n132 = case shown="False" w301 {
                  tunnel: w300 -> [_ w314]
                  tunnel: [w313 w314] -> w299
                  frame False {
                    n133 = local read "Error"() -> (w313:string)
                  }
                  frame True {
                  }
                }
                n134 = Bundle(cluster=w303, "source"=w299) -> (w302:errorcluster)  [unwired: 2 in]
                n135 = local write "Axes"(w310) -> ()
              }
              frame Error {
              }
            }
          }
          frame Error {
          }
        }
      }
    }
    n136 = local read "do stop"() -> (w261:bool)
    n137 = case shown="True" w261 {
      tunnel: w261 -> [w271 w275]
      tunnel: [w271 w275] -> w262
      frame False {
      }
      frame True {
        n138 = property class="App"() -> ("App.Kind"=w274:T3)  [unwired: 2 in, 2 out]
        n139 = Equal?(x=w274, y=T3."Run Time System" ("Application:Kind")) -> (x = y?=w272:bool)
        n140 = case shown="True" w272 {
          frame False {
          }
          frame True {
            n141 = Open VI Reference(vi path=path "Display.vi") -> (vi reference=w276:refnum<vi>)  [unwired: 5 in, 1 out]
            n142 = Open VI Reference(vi path=path "MultiAxisControl.vi") -> (vi reference=w278:refnum<vi>)  [unwired: 5 in, 1 out]
            n143 = invoke class="VI" method="FP.Close"(reference=w276) -> ()  [unwired: 2 in, 3 out]
            n144 = invoke class="VI" method="FP.Close"(reference=w278) -> ()  [unwired: 2 in, 3 out]
          }
        }
      }
    }
    n145 = call "ParseError.vi"("error in (no error)"=w266) -> ("error out"=w269:errorcluster)  [unwired: 10 in]
    n146 = Unbundle(w269) -> ("source"=w270:string)  [unwired: 2 out]
    n147 = local write "Error"(w270) -> ()
  }
  "Error" <- ""
  "do stop" <- "stop"
  "Status" <- ""
